vi "Flock_Shared_FGVQueueReferences.vi"(7 "Action":T4=enum."Get", 8 "error in (no error)":errorcluster, 9 "Queue Name":T3, 10 "Central Queue in":T2, 11 "Local Queue in":T2) -> (0 "error out":errorcluster, 2 "Central Queue out":T2, 3 "Array":T1)   [LabVIEW 2014, in "Flock_Shared_Messaging.lvlib"]
uses:
  Flock_Shared_Messaging.lvlib
  <vilib>/NI/AMC/Compatibility/amc_Message Queue.ctl
  ProcessList.ctl
  Backend/source/VI Source/Dependencies/Keyed Array/KeyedArray.ctl
  Backend/source/VI Source/Dependencies/Keyed Array/Tools_KeyedArray.lvlib
  Backend/source/VI Source/Dependencies/AMC/_SubVIs/TypeDefs/Message.ctl
  Backend/source/VI Source/Dependencies/AMC/AMC.lvlib
  FGV_Action.ctl
  FGV_Queues.ctl
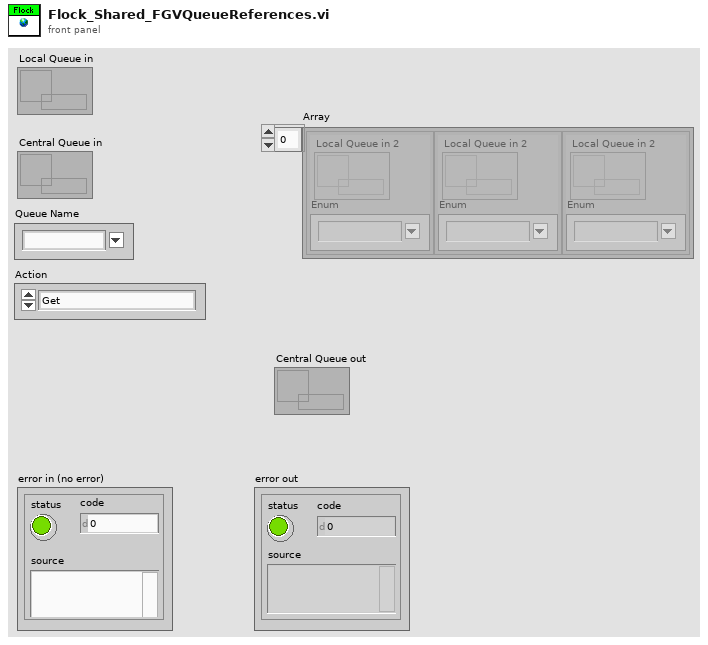
[diagram p1: front panel]
types:
  T1 = typedef "Flock_Shared_Messaging.lvlib/FGV_Queues.ctl" = cluster{"Local Queue in 2":T2, "Enum":T3}[]
  T2 = typedef "amc_Message Queue.ctl" = refnum<queue>
  T3 = typedef "Flock_Shared_Messaging.lvlib/ProcessList.ctl" = string
  T4 = typedef "FGV_Action.ctl" = enum16{"Initalize Central", "Initialize Local", "Get", "Delete Local"}
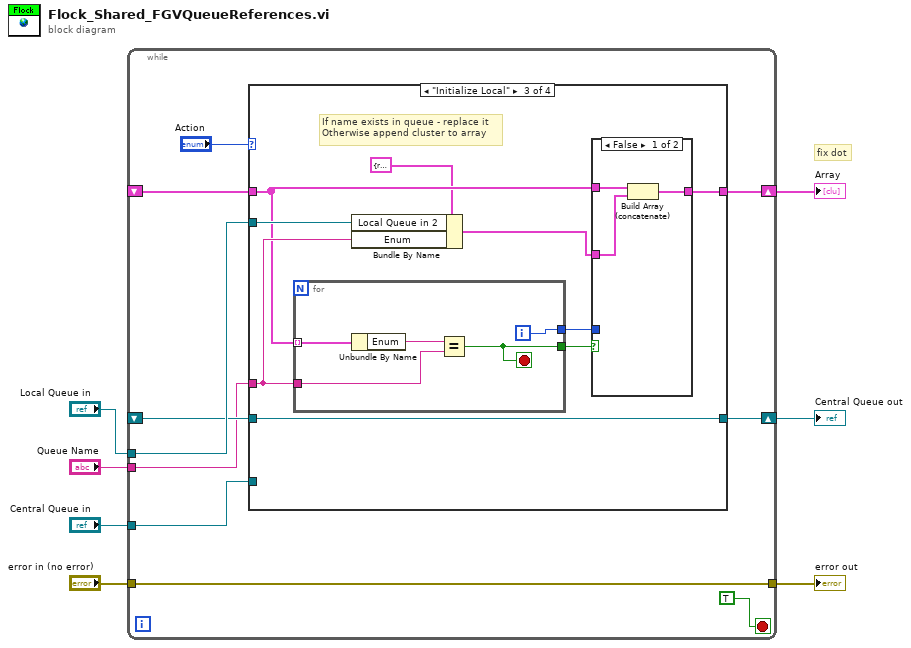
[diagram p0: block diagram]
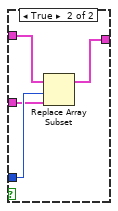
[diagram p4: hidden frame]
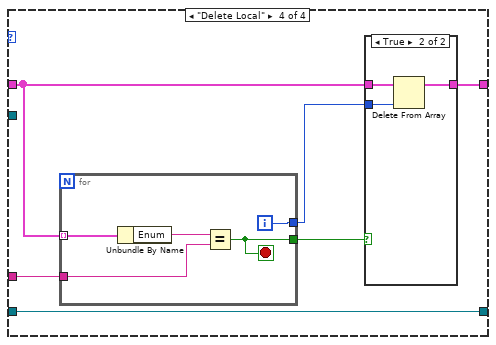
[diagram p5: hidden frame]
diagram:
  # "fix dot"
  n1 = while {
    shift-right: [w13] -> w1
    shift-left: _ -> [w14]
    tunnel: "Local Queue in" -> [w16]
    shift-right: [w12] -> w5
    shift-left: _ -> [w11]
    tunnel: "Central Queue in" -> [w10]
    tunnel: "error in (no error)" -> [w9]
    tunnel: [w9] -> w7
    tunnel: "Queue Name" -> [w8]
    stop <- TRUE ("stop") stop-if-true
    n2 = case shown="\"Initialize Local\"" "Action" {
      tunnel: [w18 w21 w23 w45] -> w13
      tunnel: w14 -> [w18 w21 w25 w46]
      tunnel: w16 -> [_ _ w29 _]
      tunnel: [w19 w20 w30 w43] -> w12
      tunnel: w11 -> [_ w20 w30 w43]
      tunnel: w10 -> [w19 _ _ _]
      tunnel: w8 -> [_ _ w28 w48]
      frame "Initalize Central" {
      }
      frame "Get" {
      }
      frame "Initialize Local" {
        # "If name exists in queue - replace it\nOtherwise append cluster to array"
        n3 = for {
          tunnel: w25 -> [w42] mode=indexing
          tunnel: w28 -> [w40]
          tunnel: [w39] -> w27
          tunnel: [w38] -> w26
          i -> [w38]
          stop <- w39 stop-if-true
          n4 = Unbundle By Name(w42) -> ("Enum"=w41:T3)
          n5 = Equal?(x=w41, y=w40) -> (x = y?=w39:bool)
        }
        n6 = Bundle By Name(cluster=cluster{"Local Queue in 2":T2, "Enum":T3} {"Local Queue in 2"=refnum, "Enum"=""} ("Cluster"), "Local Queue in 2"=w29, "Enum"=w28) -> (w22:cluster{"Local Queue in 2":T2, "Enum":T3})
        n7 = case shown="False" w27 {
          tunnel: w26 -> [_ w36]
          tunnel: w25 -> [w32 w37]
          tunnel: w22 -> [w31 w35]
          tunnel: [w33 w34] -> w23
          frame False {
            n8 = Build Array (concatenate)(w32, w31) -> (w33:cluster{"Local Queue in 2":T2, "Enum":T3}[])
          }
          frame True {
            n9 = Replace Array Subset(array=w37, new element=w35, index=w36) -> (w34:cluster{"Local Queue in 2":T2, "Enum":T3}[])
          }
        }
      }
      frame "Delete Local" {
        n10 = for {
          tunnel: w46 -> [w57] mode=indexing
          tunnel: w48 -> [w55]
          tunnel: [w54] -> w47
          tunnel: [w53] -> w44
          i -> [w53]
          stop <- w54 stop-if-true
          n11 = Unbundle By Name(w57) -> ("Enum"=w56:T3)
          n12 = Equal?(x=w56, y=w55) -> (x = y?=w54:bool)
        }
        n13 = case shown="True" w47 {
          tunnel: w46 -> [w49 w52]
          tunnel: [w49 w51] -> w45
          tunnel: w44 -> [_ w50]
          frame False {
          }
          frame True {
            n14 = Delete From Array(array=w52, index=w50) -> (array with subset deleted=w51:cluster{"Local Queue in 2":T2, "Enum":T3}[])  [unwired: 1 in, 1 out]
          }
        }
      }
    }
  }
  "Central Queue out" <- w5
  "error out" <- w7
  "Array" <- w1
